vi "Untitled 1.vi"(4 "User Parameter":T1, 5 "Event Data":cluster{"uiMsg":refnum<k7>, "cancel":bool}, 6 "Control Ref":refnum<k7>, 7 "Event Common Data":T2) -> (1 "Event Data Out":cluster{"cancel":bool})   [LabVIEW 2018]
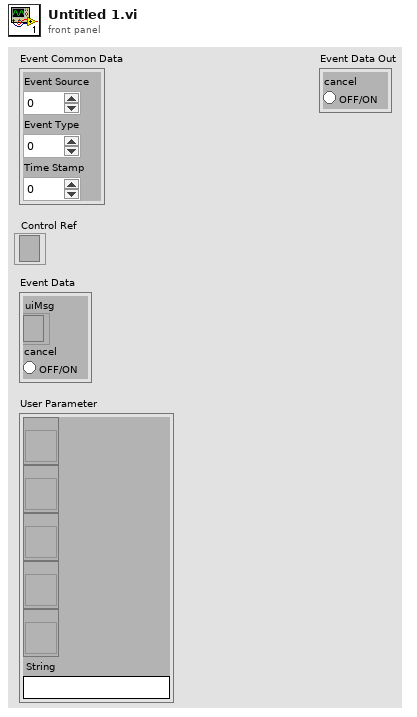
[diagram p1: front panel]
types:
  T1 = cluster{refnum<vi>, refnum<vi>, refnum<vi>, refnum<vi>, refnum<vi>, "String":string}
  T2 = cluster{"Event Source":i32, "Event Type":u32, "Time Stamp":u32}
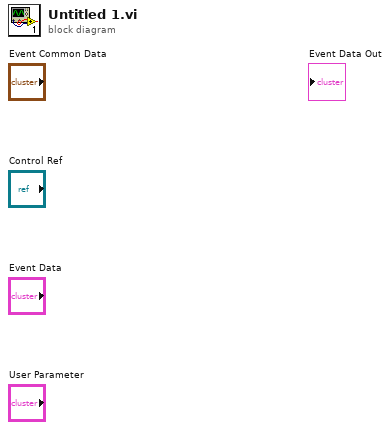
[diagram p0: block diagram]
diagram:
